vi "acceleration.vi"(7 "Max. Speed":dbl, 10 "Right":dbl, 11 "Left":dbl) -> (2 "PWM right":dbl, 3 "PWM left":dbl)   [LabVIEW 2016]
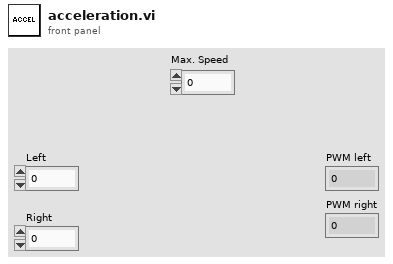
[diagram p1: front panel]
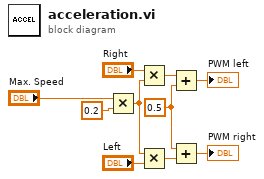
[diagram p0: block diagram]
diagram:
  w10 = 0.5 ("x")
  n1 = Multiply(x="Max. Speed", y=0.2) -> (x*y=w6:dbl)
  n2 = Multiply(x="Right", y=w6) -> (x*y=w8:dbl)
  n3 = Multiply(x=w6, y="Left") -> (x*y=w9:dbl)
  n4 = Add(x=w8, y=w10) -> (x+y=→"PWM left":dbl)
  n5 = Add(x=w10, y=w9) -> (x+y=→"PWM right":dbl)
